vi "Self-Test.vi"(8 "error in (no error)":errorcluster, 11 "Self-Test in":refnum<class "Self-Test.lvclass">) -> (0 "error out":errorcluster, 2 "Result":variant, 3 "Self-Test out":refnum<class "Self-Test.lvclass">)   [LabVIEW 2020, in "Instrument.lvlib" / "Self-Test.lvclass"]
uses:
  Self-Test.lvclass
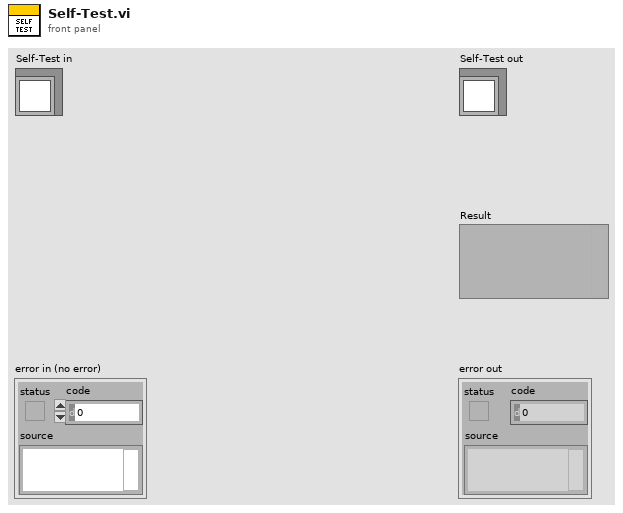
[diagram p1: front panel]
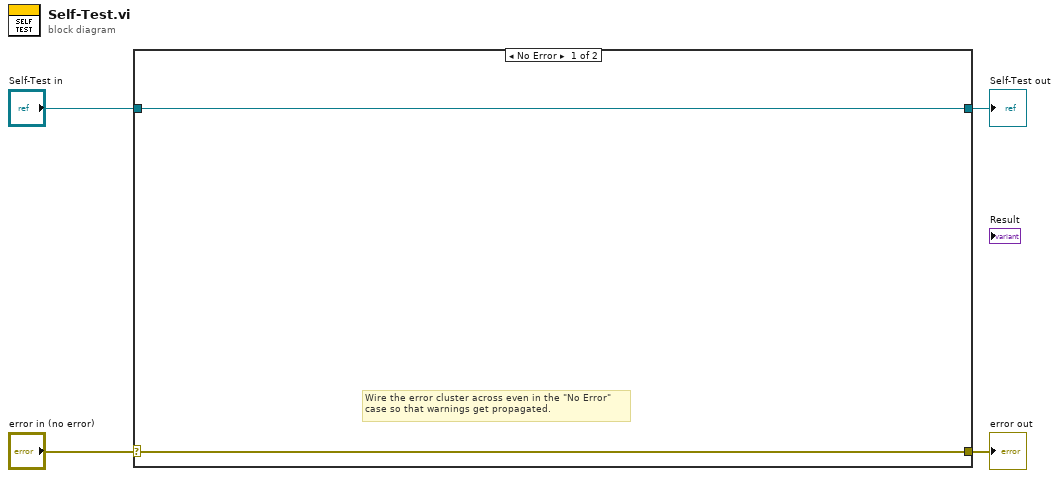
[diagram p0: block diagram]
diagram:
  n1 = case shown="No Error" "error in (no error)" {
    selector: "error in (no error)" -> [w5 w8]
    tunnel: [w5 w8] -> w3
    tunnel: [w6 w7] -> w1
    tunnel: "Self-Test in" -> [w6 w7]
    frame No Error {
      # "Wire the error cluster across even in the \"No Error\"\ncase so that warnings get propagated."
    }
    frame Error {
    }
  }
  "error out" <- w3
  "Self-Test out" <- w1
